vi "SRVDisplayChoices.vi"(6 "Delete INI File First? (F)":bool, 8 "error in (no error)":errorcluster, 11 "SRV IP Address":string) -> (0 "error out":errorcluster, 1 "Cancelled?":bool, 3 "SRV IP Address out":string)   [LabVIEW 2009]
doc: "Modified for Benilde St. Margaret's School - Tim Jump\nBy Doug Schmertman, Mike Schultz - Logic PD\nCopyright 2012"
uses:
  <vilib>/Utility/config.llb/Write Key (String).vi
  <vilib>/Utility/config.llb/NI_LVConfig.lvlib
panel:
  in  "Panes":enum32{"Table", "Add one"}(tab)
  in  "Cancel Connect":bool
  in  "Remove":bool
  in  "History":i32(listbox)
  in  "Done":bool
  in  "Add":bool
  in  "IP Address":string
  in  "Name":string
  in  "Add to list":bool
  in  "Cancel":bool
  in  "Test":bool
  # "Listed below are the previously used IP addresses.\nTo add your own, press the \"Add...\" button.  To test the connection, double click on the name."
  # "This LabVIEW item is deprecated.\n\nIt is believed to be unused and will be removed in a future version of SRV."
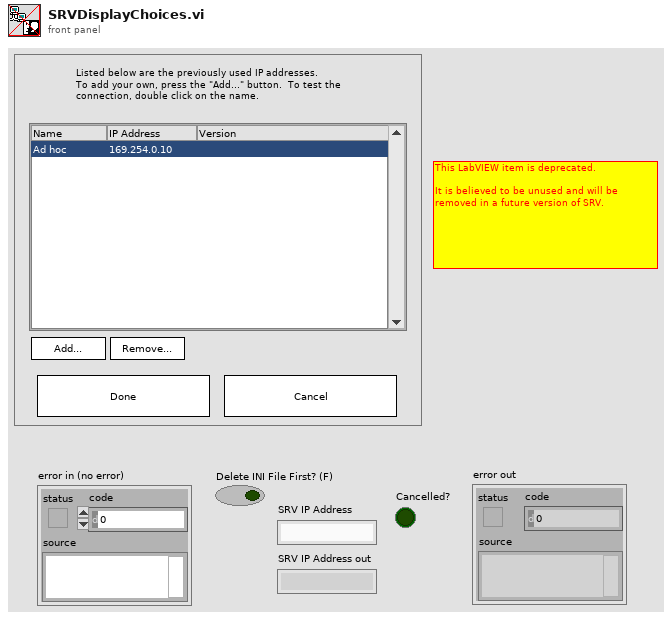
[diagram p1: front panel]
types:
  T1 = typedef "NI_LVConfig.lvlib/Config Data RefNum.ctl" = refnum<k1>
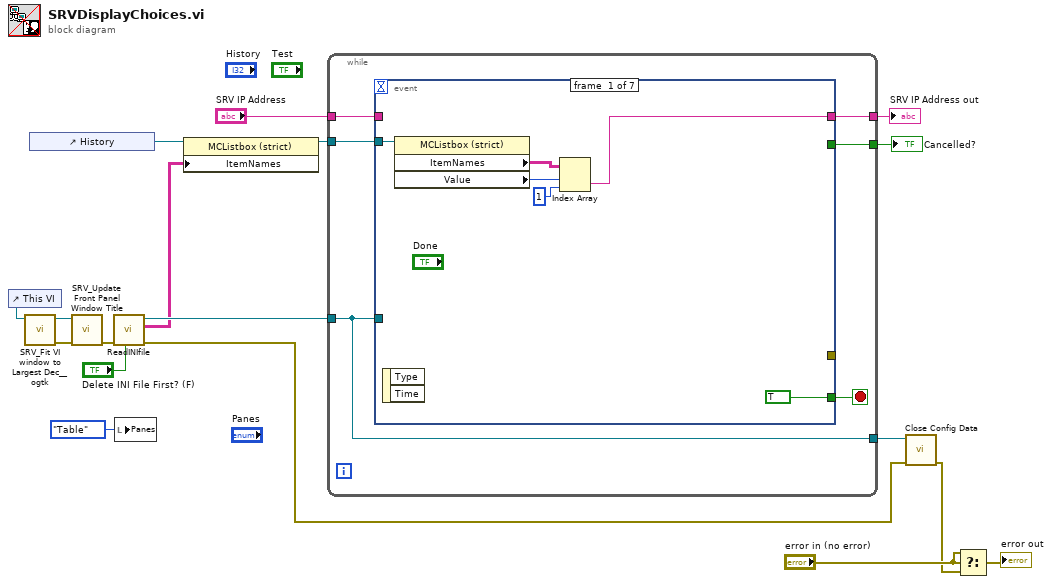
[diagram p0: block diagram]
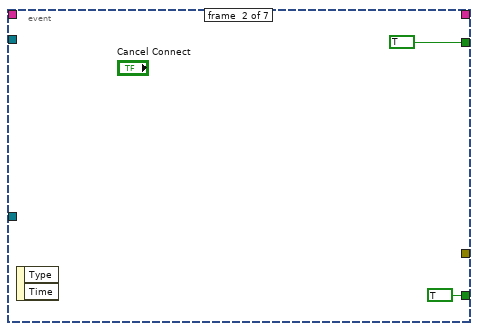
[diagram p2: hidden frame]
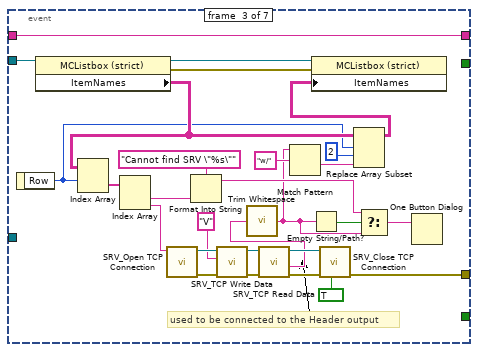
[diagram p3: hidden frame]
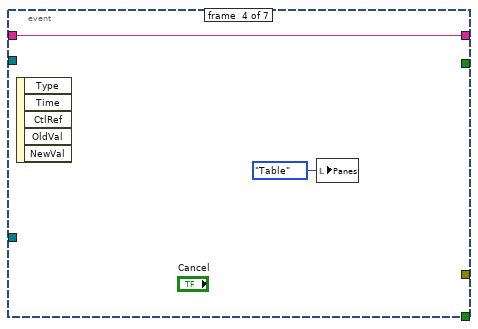
[diagram p4: hidden frame]
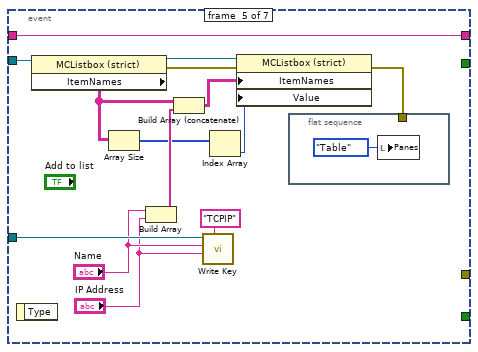
[diagram p5: hidden frame]
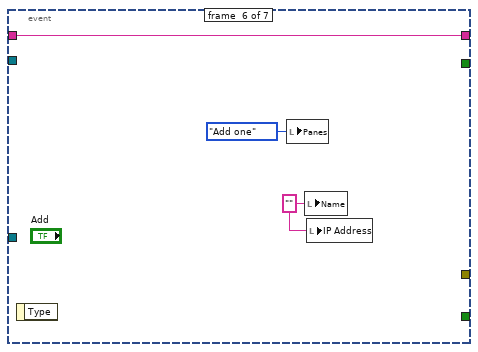
[diagram p6: hidden frame]
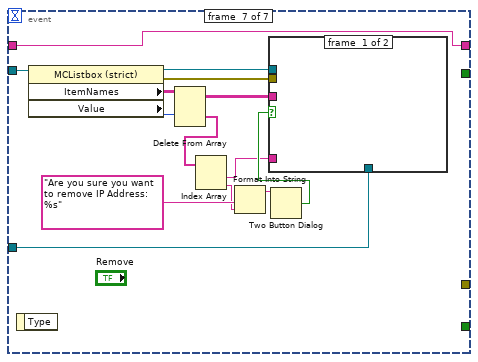
[diagram p7: hidden frame]
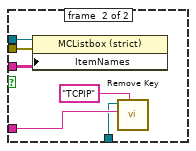
[diagram p8: hidden frame]
diagram:
  n1 = control-ref of="This VI"() -> (w6:refnum<vi>)
  n2 = call "SRV_Fit VI window to Largest Dec__ogtk.vi"("VI Ref (calling VI)"=w6) -> ("error out"=w4:errorcluster, "dup VI Ref"=w5:refnum<vi>)  [unwired: 5 in]
  n3 = control-ref of="History"() -> (w15:refnum<vi>)
  n4 = call "SRV_Update Front Panel Window Title.vi"("error in (no error)"=w4, "VI ref"=w5) -> ("error out"=w3:errorcluster)  [unwired: 8 in, 1 out]
  n5 = call "ReadINIfile.vi"("Delete INI File First? (F)"="Delete INI File First? (F)", "error in (no error)"=w3) -> ("error out"=w10:errorcluster, "Existing Addresses"=w11:string[][], "refnum out"=w12:T1)  [unwired: 7 in]
  n6 = local write "Panes"(enum32{"Table", "Add one"}."Table" ("Panes")) -> ()
  n7 = property class="MCListbox (strict)"(reference=w15, "ItemNames"=w11) -> (reference out=w14:refnum<vi>)  [unwired: 1 in, 1 out]
  n8 = while {
    tunnel: w14 -> [w23]
    tunnel: [w22] -> w17
    tunnel: "SRV IP Address" -> [w21]
    tunnel: [w20] -> w13
    tunnel: w12 -> [w20]
    tunnel: [w19] -> w2
    stop <- w24 stop-if-true
    n9 = event shown="[2] \"History\": Double Click" {
      selector: _ -> [_ _ _ _ _ _ _]
      dyn-events: _ -> [_ _ _ _ _ _ _]
      timeout: _ -> [_ _ _ _ _ _ _]
      tunnel: [TRUE ("Done") TRUE ("Done") _ _ _ _ _] -> w24
      tunnel: [_ _ w51 _ _ _ _] -> _
      tunnel: w23 -> [w27 _ w50 _ w74 _ w92]
      tunnel: [w25 _ w49 w61 w72 w79 w84] -> w22
      tunnel: w21 -> [_ _ w49 w61 w72 w79 w84]
      tunnel: w20 -> [_ _ _ _ w65 _ w82]
      tunnel: [_ TRUE ("Cancel Connect") _ _ _ _ _] -> w19
      event #0 {
        n10 = event-data() -> ()  [unwired: 1 in, 2 out]
        n11 = property class="MCListbox (strict)"(reference=w27) -> ("ItemNames"=w28:string[][], "Value"=w26:i32)  [unwired: 1 in, 2 out]
        n12 = Index Array(array=w28, index (row)=w26, index (col)=1 ("disabled index (col)")) -> (element=w25:string)
      }
      event #1 {
        n13 = event-data() -> ()  [unwired: 1 in, 2 out]
      }
      event #2 {
        # "used to be connected to the Header output"
        n14 = event-data() -> ("Row"=w36:i32)  [unwired: 1 in]
        n15 = property class="MCListbox (strict)"(reference=w50) -> (reference out=w59:refnum<vi>, error out=w58:errorcluster, "ItemNames"=w38:string[][])  [unwired: 1 in]
        n16 = Index Array(array=w38, index (row)=w36) -> (element=w44:string[])  [unwired: 1 in]
        n17 = Index Array(array=w44) -> (element #1=w42:string, element #2=w43:string)  [unwired: 2 in]
        n18 = call "SRV_Open TCP Connection.vi"("IP address"=w43) -> ("error out"=w54:errorcluster, "connection ID"=w55:refnum<k5>)  [unwired: 9 in]
        n19 = Format Into String(format string="Cannot find SRV \"%s\"" ("regular expression"), w42) -> (resulting string=w40:string)  [unwired: 2 in, 1 out]
        n20 = call "SRV_TCP Write Data.vi"("error in"=w54, "data in"="V", "connection ID"=w55) -> ("error out"=w56:errorcluster, "connection ID out"=w57:refnum<k5>)  [unwired: 6 in, 1 out]
        n21 = call "SRV_TCP Read Data.vi"("error in"=w56, "connection ID in"=w57) -> ("error out"=w39:errorcluster, "data out"=w33:string, "connection ID"=w53:refnum<k5>)  [unwired: 3 in, 1 out]
        n22 = call <vilib>:"Trim Whitespace.vi"("string"=w33) -> ("trimmed string"=w35:string)  [unwired: 1 in]
        n23 = Match Pattern(string=w35, regular expression="w/") -> (after substring=w48:string)  [unwired: 1 in, 3 out]
        n24 = Empty String/Path?(string/path=w35) -> (empty?=w46:bool)
        n25 = call "SRV_Close TCP Connection.vi"("Force Reset? (F)"=TRUE, "error in"=w39, "connection ID"=w53) -> ("error out"=w51:errorcluster)  [unwired: 8 in]
        n26 = Replace Array Subset(array=w38, new element=w48, index (row)=w36, index (col)=2 ("disabled index (col)")) -> (w37:string[][])
        n27 = property class="MCListbox (strict)"(reference=w59, error in=w58, "ItemNames"=w37) -> ()  [unwired: 2 out]
        n28 = Select(t=w40, s=w46, f=w35) -> (s? t:f=w45:string)
        n29 = One Button Dialog(message=w45) -> ()  [unwired: 1 in, 1 out]
      }
      event #3 {
        n30 = event-data() -> ()  [unwired: 1 in, 5 out]
        n31 = local write "Panes"(enum32{"Table", "Add one"}."Table" ("Panes")) -> ()
      }
      event #4 {
        n32 = event-data() -> ()  [unwired: 1 in, 1 out]
        n33 = property class="MCListbox (strict)"(reference=w74) -> (reference out=w76:refnum<vi>, error out=w75:errorcluster, "ItemNames"=w71:string[][])  [unwired: 1 in]
        n34 = Array Size(array=w71) -> (size(s)=w70:i32[])
        n35 = Build Array("Name", "IP Address") -> (w73:string[])
        n36 = Build Array (concatenate)(w71, w73) -> (w67:string[][])
        n37 = call-poly <vilib>:"Write Key.vi"("section"="TCPIP", "value"="IP Address", "key"="Name", "refnum"=w65) -> ()  [unwired: 5 in, 3 out]
        n38 = Index Array(array=w70) -> (element=w69:i32)  [unwired: 1 in]
        n39 = property class="MCListbox (strict)"(reference=w76, error in=w75, "ItemNames"=w67, "Value"=w69) -> (error out=w68:errorcluster)  [unwired: 1 out]
        n40 = flat-sequence {
          tunnel: w68 -> [_]
          frame #0 {
            n41 = local write "Panes"(enum32{"Table", "Add one"}."Table" ("Panes")) -> ()
          }
        }
      }
      event #5 {
        w78 = "" ("Name")
        n42 = event-data() -> ()  [unwired: 1 in, 1 out]
        n43 = local write "Panes"(enum32{"Table", "Add one"}."Add one" ("Panes")) -> ()
        n44 = local write "Name"(w78) -> ()
        n45 = local write "IP Address"(w78) -> ()
      }
      event #6 {
        n46 = event-data() -> ()  [unwired: 1 in, 1 out]
        n47 = property class="MCListbox (strict)"(reference=w92) -> (reference out=w94:refnum<vi>, error out=w93:errorcluster, "ItemNames"=w91:string[][], "Value"=w90:i32)  [unwired: 1 in]
        n48 = Delete From Array(array=w91, index (row)=w90) -> (deleted portion=w81:string[], array with subset deleted=w89:string[][])  [unwired: 2 in]
        n49 = Index Array(array=w81) -> (element #1=w83:string, element #2=w87:string)  [unwired: 2 in]
        n50 = Format Into String(format string="Are you sure you want to remove IP Address: %s", w87) -> (resulting string=w86:string)  [unwired: 2 in, 1 out]
        n51 = Two Button Dialog(message=w86) -> (T button?=w85:bool)  [unwired: 2 in]
        n52 = case shown="True" w85 {
          tunnel: w94 -> [_ w100]
          tunnel: w93 -> [_ w99]
          tunnel: w89 -> [_ w98]
          tunnel: w83 -> [_ w97]
          tunnel: w82 -> [_ w96]
          frame #0 {
          }
          frame #1 {
            n53 = property class="MCListbox (strict)"(reference=w100, error in=w99, "ItemNames"=w98) -> ()  [unwired: 2 out]
            n54 = call <vilib>:"Remove Key.vi"("section"="TCPIP", "key"=w97, "refnum"=w96) -> ()  [unwired: 6 in, 3 out]
          }
        }
      }
    }
  }
  "SRV IP Address out" <- w17
  "Cancelled?" <- w2
  n55 = call <vilib>:"Close Config Data.vi"("error in (no error)"=w10, "refnum"=w13) -> ("error out"=w8:errorcluster)  [unwired: 8 in, 1 out]
  n56 = Select(t="error in (no error)", s="error in (no error)", f=w8) -> (s? t:f=→"error out":errorcluster)
